vi "Parse Response JSON.vi"(8 "error in (no error)":errorcluster, 10 "Response JSON":string, 11 "RGetInputVolume in":refnum<class "RGetInputVolume.lvclass">) -> (0 "error out":errorcluster, 3 "RGetInputVolume out":refnum<class "RGetInputVolume.lvclass">)   [LabVIEW 2022 SP3, in "obs-websocket-lv.lvlib" / "RGetInputVolume.lvclass"]
uses:
  RGetInputVolume.lvclass
  RGetInputVolume.lvclass/RGetInputVolume.ctl
  <vilib>/IlluminatedG/lv-web-crypto/lv-json/JSON/JSON.lvlib
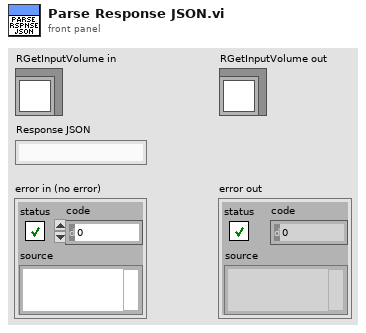
[diagram p1: front panel]
types:
  T1 = typedef "JSON.lvlib/JSON Item Type.ctl" = enum16{"unknown", "null", "Array", "Object", "String", "Number", "Boolean"}
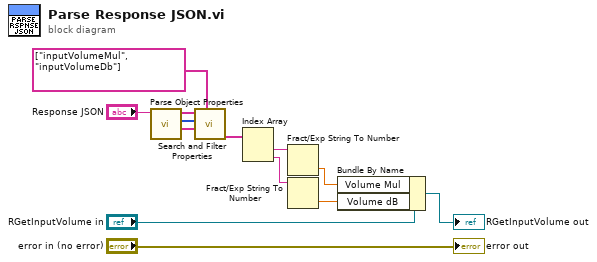
[diagram p0: block diagram]
diagram:
  n1 = call <vilib>:"Parse Object Properties.vi"("JSON String"="Response JSON") -> ("Values"=w8:string[], "Item Types"=w9:T1[], "Keys"=w10:string[])  [unwired: 7 in, 1 out]
  n2 = call <vilib>:"Search and Filter Properties.vi"("Search Keys"=string[] ["inputVolumeMul", "inputVolumeDb"], "Values In"=w8, "Types In"=w9, "Keys In"=w10) -> ("Filtered Values"=w6:string[])  [unwired: 2 in, 5 out]
  n3 = Index Array(array=w6) -> (element #1=w4:string, element #2=w5:string)  [unwired: 2 in]
  n4 = Fract/Exp String To Number(string=w4) -> (number=w2:dbl)  [unwired: 3 in, 1 out]
  n5 = Fract/Exp String To Number(string=w5) -> (number=w1:dbl)  [unwired: 3 in, 1 out]
  n6 = Bundle By Name(cluster="RGetInputVolume in", "Volume Mul"=w2, "Volume dB"=w1) -> (→"RGetInputVolume out":refnum<class "RGetInputVolume.lvclass">)
  "error out" <- "error in (no error)"
